vi "Move_2_axis_linear_Peregrine.vi"(0 "Handle in":refnum<visa-resource-name>, 1 "Address x":u8, 3 "Address y":u8, 5 "Target x":i32, 9 "Target y":i32, 11 "error":errorcluster, 12 "Speed":i16, 14 "Acceleration":u16) -> (4 "Handle out":refnum<visa-resource-name>, 15 "error out":errorcluster)   [LabVIEW 2019]
panel:
  out "dx":i32
  out "dy":i32
  out "Position y":i32
  out "Position x":i32
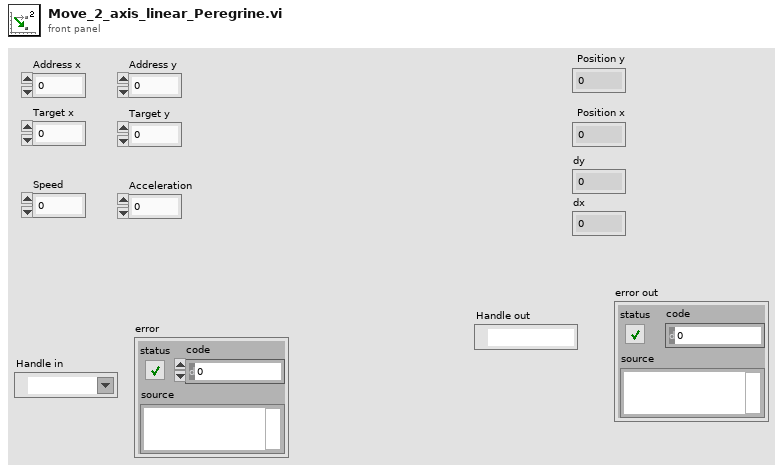
[diagram p1: front panel]
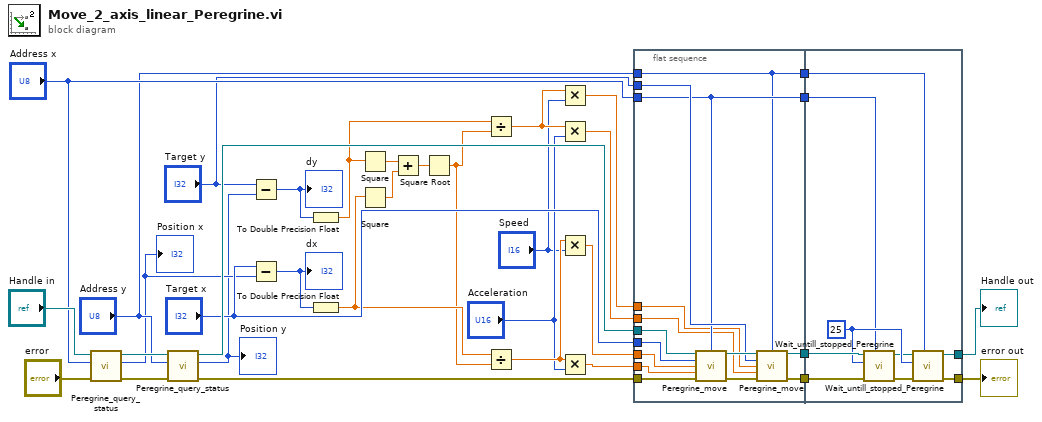
[diagram p0: block diagram]
diagram:
  n1 = call "Peregrine_query_status.vi"("error"="error", "Address"="Address x", "Handle in"="Handle in") -> ("error out"=w25:errorcluster, "Position"=w19:i32, "Handle out"=w26:refnum<visa-resource-name>)  [unwired: 4 in, 2 out]
  "Position x" <- w19
  n2 = call "Peregrine_query_status.vi"("error"=w25, "Address"="Address y", "Handle in"=w26) -> ("error out"=w28:errorcluster, "Position"=w18:i32, "Handle out"=w27:refnum<visa-resource-name>)  [unwired: 4 in, 2 out]
  "Position y" <- w18
  n3 = Subtract(x="Target y", y=w18) -> (x-y=w15:i32)
  "dy" <- w15
  n4 = Subtract(x="Target x", y=w19) -> (x-y=w16:i32)
  "dx" <- w16
  n5 = To Double Precision Float(number=w15) -> (double precision float=w9:dbl)
  n6 = To Double Precision Float(number=w16) -> (double precision float=w11:dbl)
  n7 = Square(x=w9) -> (x^2=w13:dbl)
  n8 = Square(x=w11) -> (x^2=w14:dbl)
  n9 = Add(x=w13, y=w14) -> (x+y=w12:dbl)
  n10 = Square Root(x=w12) -> (sqrt(x)=w10:dbl)
  n11 = Divide(x=w9, y=w10) -> (x/y=w7:dbl)
  n12 = Divide(x=w11, y=w10) -> (x/y=w5:dbl)
  n13 = Multiply(x=w7, y="Speed") -> (x*y=w6:dbl)
  n14 = Multiply(x=w7, y="Acceleration") -> (x*y=w8:dbl)
  n15 = Multiply(x=w5, y="Speed") -> (x*y=w2:dbl)
  n16 = Multiply(x=w5, y="Acceleration") -> (x*y=w1:dbl)
  n17 = flat-sequence {
    tunnel: "Address x" -> [w40]
    tunnel: w27 -> [w48]
    tunnel: w28 -> [w47]
    tunnel: "Target x" -> [w46]
    tunnel: [w43] -> w34
    tunnel: [w42] -> w33
    tunnel: "Target y" -> [w41]
    tunnel: [w40] -> w30
    tunnel: "Address y" -> [w39]
    tunnel: [w39] -> w29
    tunnel: w8 -> [w38]
    tunnel: w6 -> [w37]
    tunnel: w2 -> [w36]
    tunnel: w1 -> [w35]
    tunnel: w34 -> [w57]
    tunnel: w33 -> [w56]
    tunnel: [w52] -> w32
    tunnel: [w51] -> w31
    tunnel: w30 -> [w50]
    tunnel: w29 -> [w49]
    frame #0 {
      n18 = call "Peregrine_move.vi"("Handle in"=w48, "Address"=w40, "Target"=w46, "Speed"=w36, "Acceleration"=w35, "error"=w47) -> ("Handle out"=w45:refnum<visa-resource-name>, "error out"=w44:errorcluster)  [unwired: 8 in]
      n19 = call "Peregrine_move.vi"("Handle in"=w45, "Address"=w39, "Target"=w41, "Speed"=w37, "Acceleration"=w38, "error"=w44) -> ("Handle out"=w43:refnum<visa-resource-name>, "error out"=w42:errorcluster)  [unwired: 8 in]
    }
    frame #1 {
      w55 = u32 25 ("milliseconds to wait")
      n20 = call "Wait_untill_stopped_Peregrine.vi"("Address"=w50, "error"=w56, "milliseconds to wait"=w55, "Handle in"=w57) -> ("error out"=w53:errorcluster, "Handle out"=w54:refnum<visa-resource-name>)  [unwired: 2 in, 4 out]
      n21 = call "Wait_untill_stopped_Peregrine.vi"("Address"=w49, "error"=w53, "milliseconds to wait"=w55, "Handle in"=w54) -> ("error out"=w51:errorcluster, "Handle out"=w52:refnum<visa-resource-name>)  [unwired: 2 in, 4 out]
    }
  }
  "Handle out" <- w32
  "error out" <- w31
